vi "Determine If Belongs In Sector and Accumulate.vi"(6 "Left Sector Parameters":T2, 7 "Right Sector Parameters":T2, 8 "error in (no error)":errorcluster, 9 "Midpoint of Image":dbl, 10 "Starting Y Location":i32, 11 "Image Data":u8[][](array[numeric])) -> (0 "error out":errorcluster, 2 "Canceled?":bool, 3 "[Accumulated Sectors]":T1[](array[typedef]))   [LabVIEW 2013]
uses:
  FPGA/Sector/Accumulate/Sector Parameter Cluster.ctl
  FPGA/Sector/Accumulate/Accumulated Sector Cluster.ctl
panel:
  in  "Cancel Button":bool
  out "Progress":u16(slide) scale=0.0..788.0
  # "Calculating Average Sector Background ..."
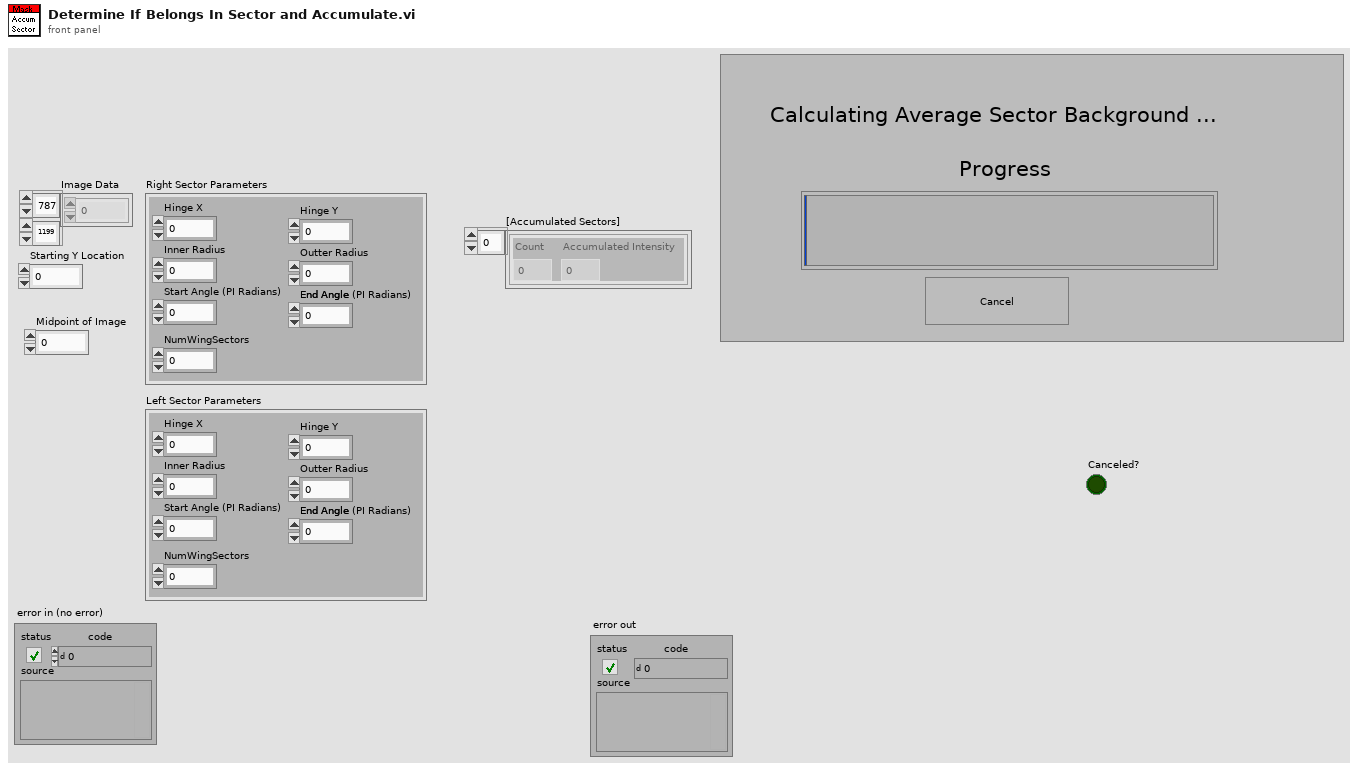
[diagram p1: front panel]
types:
  T1 = typedef "Accumulated Sector Cluster.ctl" = cluster{"Accumulated Intensity":u32, "Count":u16}
  T2 = typedef "Sector Parameter Cluster.ctl" = cluster{"Start Angle":fxp<+/-,17,2>, "End Angle":fxp<+,17,3>, "Inner Radius":u16, "Outter Radius":u16, "Hinge X":u16, "Hinge Y":u16, "NumWingSectors":u8}
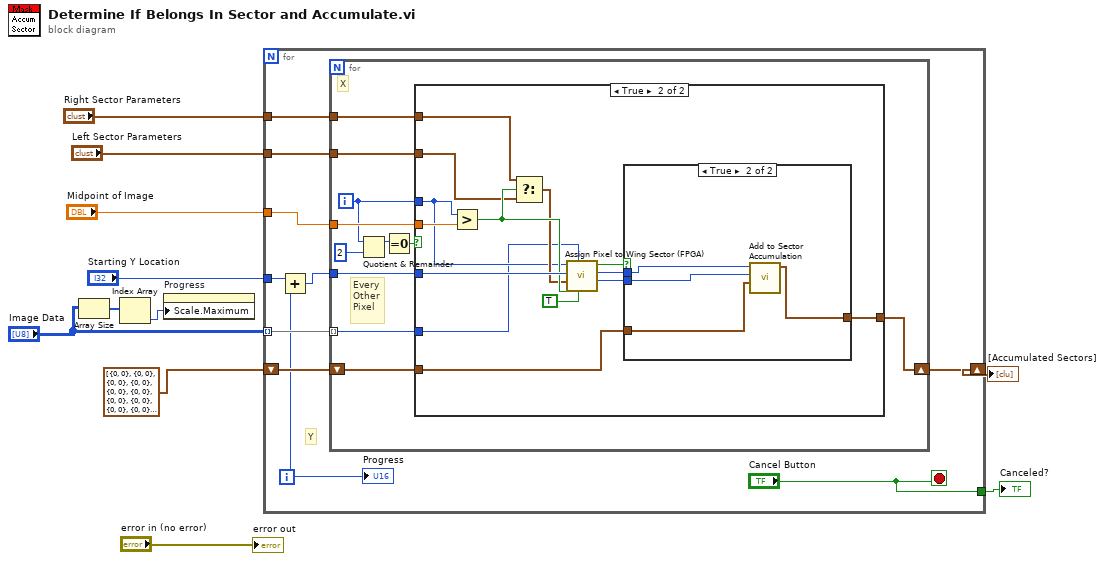
[diagram p0: block diagram]
diagram:
  n1 = Array Size(array="Image Data") -> (size(s)=w3:i32[])
  n2 = Index Array(array=w3) -> (element=w2:i32)  [unwired: 1 in]
  n3 = property on="Progress" class="Slide (strict)"("Scale.Maximum"=w2) -> ()  [unwired: 2 in, 2 out]
  n4 = for {
    tunnel: "Image Data" -> [w21] mode=indexing
    tunnel: "Midpoint of Image" -> [w20]
    tunnel: "Right Sector Parameters" -> [w19]
    tunnel: "Left Sector Parameters" -> [w18]
    shift-right: [w16] -> w6
    shift-left: T1[] [{"Accumulated Intensity"=0, "Count"=0}, {"Accumulated Intensity"=0, "Count"=0}, {"Accumulated Intensity"=0, "Count"=0}, {"Accumulated Intensity"=0, "Count"=0}, {"Accumulated Intensity"=0, "Count"=0}, {"Accumulated Intensity"=0, "Count"=0}, {"Accumulated Intensity"=0, "Count"=0}, {"Accumulated Intensity"=0, "Count"=0}, {"Accumulated Intensity"=0, "Count"=0}, {"Accumulated Intensity"=0, "Count"=0}, {"Accumulated Intensity"=0, "Count"=0}, {"Accumulated Intensity"=0, "Count"=0}, {"Accumulated Intensity"=0, "Count"=0}, {"Accumulated Intensity"=0, "Count"=0}, {"Accumulated Intensity"=0, "Count"=0}, {"Accumulated Intensity"=0, "Count"=0}, {"Accumulated Intensity"=0, "Count"=0}, {"Accumulated Intensity"=0, "Count"=0}, {"Accumulated Intensity"=0, "Count"=0}, {"Accumulated Intensity"=0, "Count"=0}, {"Accumulated Intensity"=0, "Count"=0}, {"Accumulated Intensity"=0, "Count"=0}, {"Accumulated Intensity"=0, "Count"=0}, {"Accumulated Intensity"=0, "Count"=0}, {"Accumulated Intensity"=0, "Count"=0}, {"Accumulated Intensity"=0, "Count"=0}, {"Accumulated Intensity"=0, "Count"=0}, {"Accumulated Intensity"=0, "Count"=0}, {"Accumulated Intensity"=0, "Count"=0}, {"Accumulated Intensity"=0, "Count"=0}, {"Accumulated Intensity"=0, "Count"=0}, {"Accumulated Intensity"=0, "Count"=0}] ("[Accumulated Sectors] Out") -> [w17]
    tunnel: "Starting Y Location" -> [w14]
    tunnel: ["Cancel Button"] -> w1
    i -> [w13]
    stop <- "Cancel Button" stop-if-true
    # "Y"
    n5 = Add(x=w14, y=w13) -> (x+y=w15:i32)
    n6 = for {
      tunnel: w21 -> [w28] mode=indexing
      tunnel: w15 -> [w32]
      tunnel: w20 -> [w31]
      tunnel: w19 -> [w30]
      tunnel: w18 -> [w29]
      shift-right: [w26] -> w16
      shift-left: w17 -> [w27]
      i -> [w25]
      # "Every\nOther\nPixel"
      # "X"
      n7 = Quotient & Remainder(x=w25, y=2) -> (x-y*floor(x/y)=w23:i32)  [unwired: 1 out]
      n8 = Equal To 0?(x=w23) -> (x = 0?=w22:bool)
      n9 = case shown="True" w22 {
        tunnel: w32 -> [_ w47]
        tunnel: w31 -> [_ w46]
        tunnel: w30 -> [_ w44]
        tunnel: w29 -> [_ w43]
        tunnel: w25 -> [_ w41]
        tunnel: w28 -> [_ w40]
        tunnel: w27 -> [w33 w38]
        tunnel: [w33 w36] -> w26
        frame False {
        }
        frame True {
          n10 = Greater?(x=w41, y=w46) -> (0:w45:bool)
          n11 = Select(t=w44, s=w45, f=w43) -> (s? t:f=w42:T2)
          n12 = call "Assign Pixel to Wing Sector (FPGA).vi"("Valid Data?"=TRUE, "Pixel Intensity In"=w40, "Right Wing?"=w45, "Sector Parameters"=w42, "Pixel Y"=w47, "Pixel X"=w41) -> ("Pixel Intensity Out"=w35:u8, "sector #"=w37:u8, "output valid"=w39:bool)  [unwired: 1 in, 2 out]
          n13 = case shown="True" w39 {
            tunnel: w38 -> [w48 w50]
            tunnel: w37 -> [_ w52]
            tunnel: [w48 w49] -> w36
            tunnel: w35 -> [_ w51]
            frame False {
            }
            frame True {
              n14 = call "Add to Sector Accumulation.vi"("[Accumulated Sectors] In"=w50, "Pixel Intensity"=w51, "Sector ID"=w52) -> ("[Accumulated Sectors] Out"=w49:T1[])  [unwired: 8 in]
            }
          }
        }
      }
    }
    "Progress" <- w13
  }
  "[Accumulated Sectors]" <- w6
  "Canceled?" <- w1
  "error out" <- "error in (no error)"
